vi "Get Saving Data.vi"(8 "Ordinal":i32, 9 "Measure_No":i32, 10 "Left Or Right":string, 11 "Measure_ID":i32) -> (2 "Get Saving Data Path":T2, 3 "Biometry Attribute":T1)   [LabVIEW 2015, in "Utility VIs.lvlib"]
uses:
  Utility VIs.lvlib
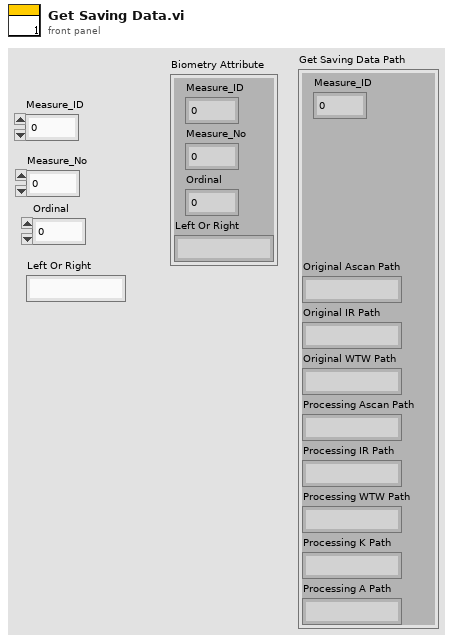
[diagram p1: front panel]
types:
  T1 = cluster{"Measure_ID":i32, "Measure_No":i32, "Ordinal":i32, "Left Or Right":string}
  T2 = cluster{"Measure_ID":i32, "Original Ascan Path":string, "Original IR Path":string, "Original WTW Path":string, "Processing Ascan Path":string, "Processing IR Path":string, "Processing WTW Path":string, "Processing K Path":string, "Processing A Path":string}
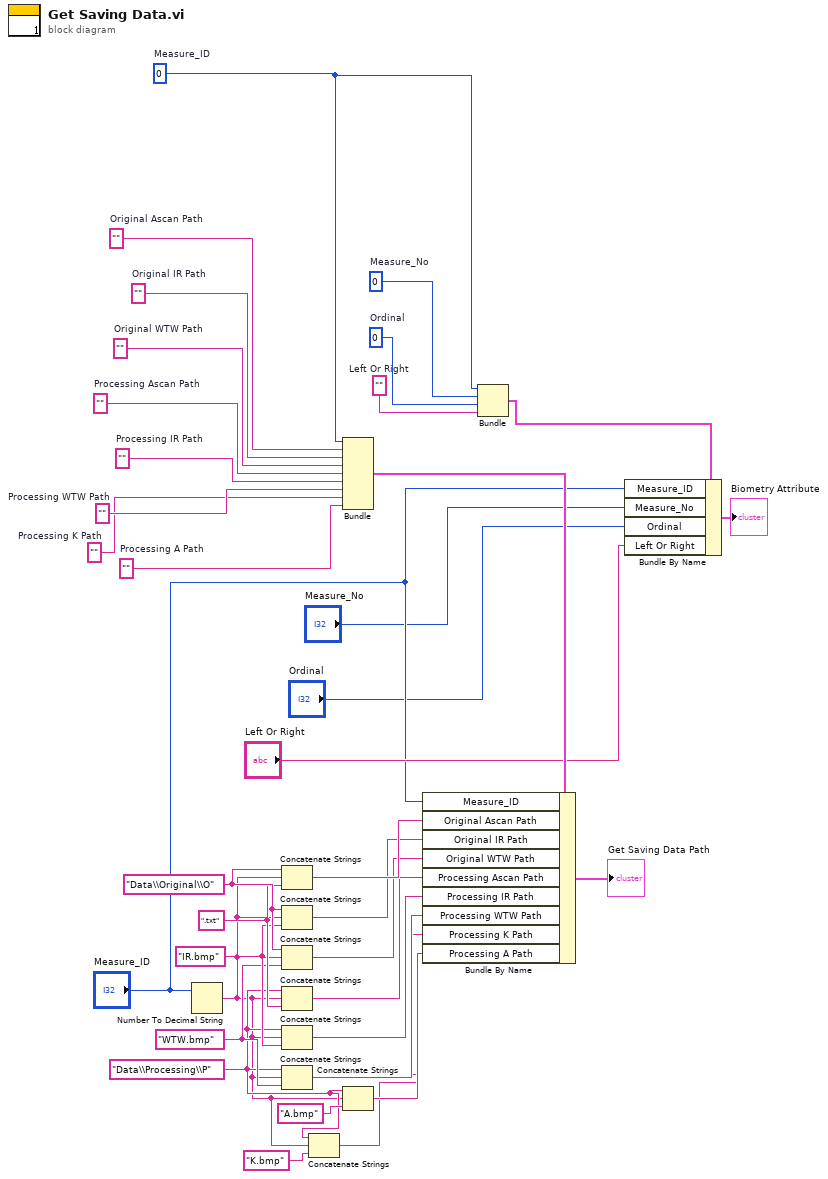
[diagram p0: block diagram]
diagram:
  w16 = ""  # Processing K Path
  w11 = 0  # Measure_ID
  w10 = 0  # Measure_No
  w9 = 0  # Ordinal
  w8 = ""  # Left Or Right
  w25 = ""  # Processing A Path
  w26 = ""  # Processing WTW Path
  w27 = ""  # Processing IR Path
  w28 = ""  # Processing Ascan Path
  w29 = ""  # Original WTW Path
  w30 = ""  # Original IR Path
  w31 = ""  # Original Ascan Path
  w14 = "Data\\Processing\\P"
  w33 = "WTW.bmp" ("字符串")
  w34 = "IR.bmp" ("字符串")
  w35 = ".txt" ("字符串")
  w36 = "Data\\Original\\O"
  n1 = Number To Decimal String(number="Measure_ID") -> (decimal integer string=w13:string)  [unwired: 1 in]
  n2 = Concatenate Strings(w36, w13, w35) -> (w23:string)
  n3 = Concatenate Strings(w36, w13, w34) -> (w22:string)
  n4 = Concatenate Strings(w36, w13, w33) -> (w21:string)
  n5 = Concatenate Strings(w14, w13, w35) -> (w20:string)
  n6 = Concatenate Strings(w14, w13, w34) -> (w19:string)
  n7 = Concatenate Strings(w14, w13, w33) -> (w18:string)
  n8 = Concatenate Strings(w14, w13, "K.bmp" ("字符串")) -> (w15:string)
  n9 = Bundle("Measure_ID"=w11, "Original Ascan Path"=w31, "Original IR Path"=w30, "Original WTW Path"=w29, "Processing Ascan Path"=w28, "Processing IR Path"=w27, "Processing WTW Path"=w26, "Processing K Path"=w16, "Processing A Path"=w25) -> (w24:T2)  [unwired: 1 in]
  n10 = Concatenate Strings(w14, w13, "A.bmp" ("字符串")) -> (w17:string)
  n11 = Bundle By Name(cluster=w24, "Measure_ID"="Measure_ID", "Original Ascan Path"=w23, "Original IR Path"=w22, "Original WTW Path"=w21, "Processing Ascan Path"=w20, "Processing IR Path"=w19, "Processing WTW Path"=w18, "Processing K Path"=w15, "Processing A Path"=w17) -> (→"Get Saving Data Path":T2)
  n12 = Bundle("Measure_ID"=w11, "Measure_No"=w10, "Ordinal"=w9, "Left Or Right"=w8) -> (w7:T1)  [unwired: 1 in]
  n13 = Bundle By Name(cluster=w7, "Measure_ID"="Measure_ID", "Measure_No"="Measure_No", "Ordinal"="Ordinal", "Left Or Right"="Left Or Right") -> (→"Biometry Attribute":T1)
